vi "IBM4_Read(I1).vi"(8 "error in":errorcluster, 10 "Channel":enum16{"A2", "A3", "A4", "A5"}(ring), 11 "COM resource in":refnum<visa-resource-name>="COM9") -> (0 "error out":errorcluster, 2 "output":i32, 3 "COM resource out":refnum<visa-resource-name>)   [LabVIEW 2021, in "IBM4.lvlib"]
doc: "This VI interfaces with the IBM4 to perform a read operation.\n\nThe output will in binary format (thus, integer).\nOnly a single read operation is made with this VI. \n\nAlternate read operations exist covering binary or floating point, single reading, multiple readings, and an average of multiple readings (floating point only)."
uses:
  <instrlib>/IBM4/IBM4.lvlib
panel:
  out "read buffer":string
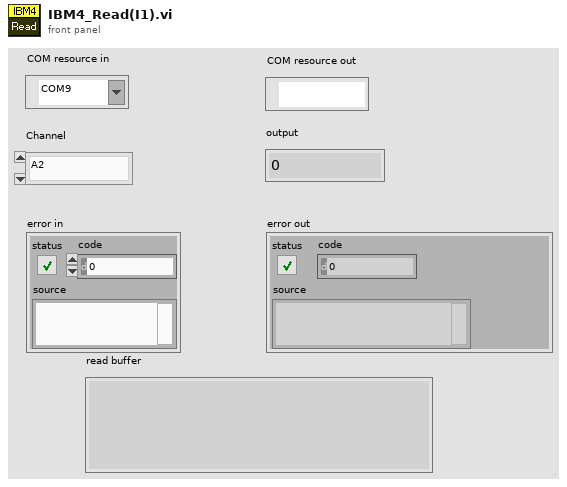
[diagram p1: front panel]
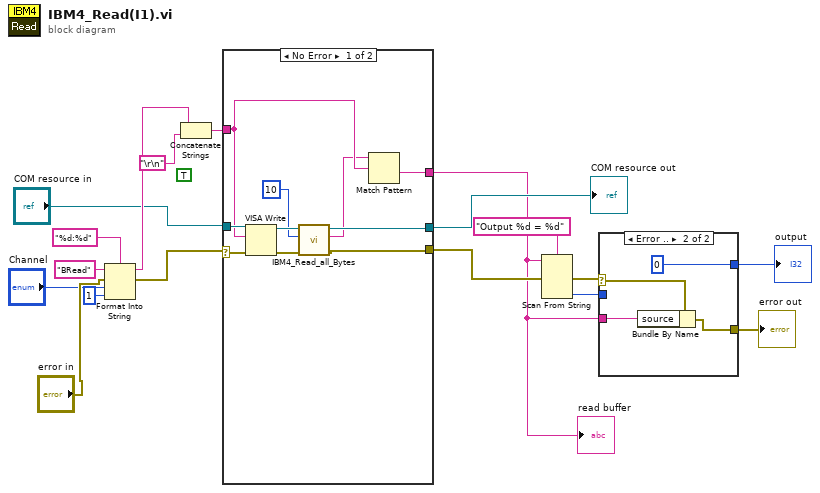
[diagram p0: block diagram]
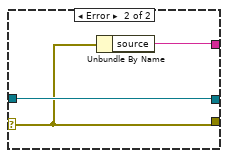
[diagram p3: hidden frame]
diagram:
  (unwired) TRUE ("Enable Termination\nChar (T)")
  n1 = Format Into String(format string="%d:%d", initial string="BRead", error in="error in", "Channel", 1 ("input 2")) -> (resulting string=w9:string, error out=w1:errorcluster)
  n2 = Concatenate Strings(w9, "\r\n") -> (w8:string)
  n3 = case shown="No Error" w1 {
    selector: w1 -> [w25 w29]
    tunnel: "COM resource in" -> [w28 w31]
    tunnel: [w21 w29] -> w12
    tunnel: [w27 w30] -> w3
    tunnel: w8 -> [w26 _]
    tunnel: [w22 w31] -> w13
    frame No Error {
      n4 = VISA Write(VISA resource name=w28, write buffer=w26, error in (no error)=w25) -> (VISA resource name out=w23:refnum<visa-resource-name>, error out=w24:errorcluster)  [unwired: 1 out]
      n5 = call <instrlib>:"IBM4_Read_all_Bytes.vi"("error in (no error)"=w24, "milliseconds to wait"=u32 10, "VISA Refnum in"=w23) -> ("error out"=w21:errorcluster, "String"=w20:string, "VISA Refnum out"=w22:refnum<visa-resource-name>)  [unwired: 2 in]
      n6 = Match Pattern(string=w20, regular expression=w26) -> (after substring=w27:string)  [unwired: 1 in, 3 out]
    }
    frame Error {
      n7 = Unbundle By Name(w29) -> ("source"=w30:string)
    }
  }
  "COM resource out" <- w13
  "read buffer" <- w3
  n8 = Scan From String(format string="Output %d = %d", input string=w3, error in=w12) -> (error out=w7:errorcluster, output 2=w6:i32)  [unwired: 4 in, 2 out]
  n9 = case shown="Error .." w7 {
    selector: w7 -> [w32 w36]
    tunnel: w6 -> [w33 _]
    tunnel: [w33 0] -> w5
    tunnel: [w32 w34] -> w4
    tunnel: w3 -> [_ w35]
    frame No Error {
    }
    frame Error {
      n10 = Bundle By Name(cluster=w36, "source"=w35) -> (w34:errorcluster)
    }
  }
  "error out" <- w4
  "output" <- w5
